vi "Build Report String.vi"(0 "folders":string[](array[string]), 5 "file paths":path[][](array[path]), 11 "error in":errorcluster) -> (4 "report string out":string, 15 "error out":errorcluster)   [LabVIEW 2019, in "MD Generator.lvlib"]
uses:
  MD Generator.lvlib
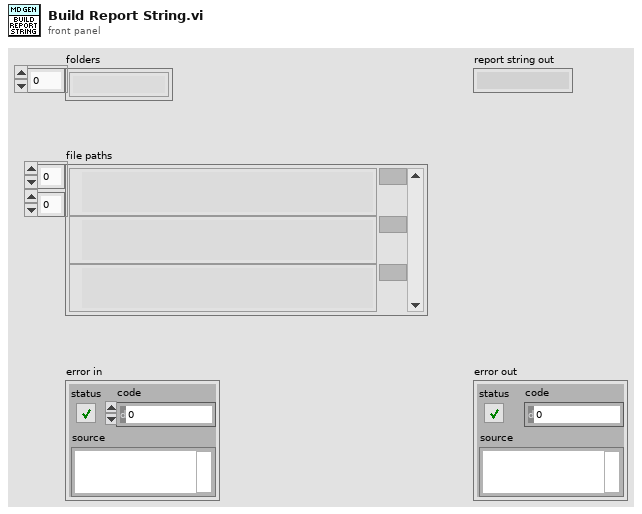
[diagram p1: front panel]
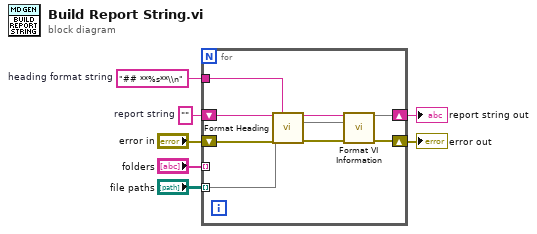
[diagram p0: block diagram]
diagram:
  w2 = ""  # report string
  w7 = "## **%s**\\n"  # heading format string
  n1 = for {
    shift-right: [w14] -> w1
    shift-left: w2 -> [w13]
    shift-right: [w12] -> w3
    shift-left: "error in" -> [w11]
    tunnel: w7 -> [w9]
    tunnel: "folders" -> [_] mode=indexing
    tunnel: "file paths" -> [w8] mode=indexing
    n2 = call "Format Heading.vi"("new heading"=w13, "format string"=w9, "error in"=w11) -> ("string out"=w10:string, "error out"=w15:errorcluster)  [unwired: 11 in]
    n3 = call "Format VI Information.vi"("filenames"=w10, 5:w8, "error in"=w15) -> (4:w14, "error out"=w12:errorcluster)  [unwired: 10 in, 1 out]
  }
  "error out" <- w3
  "report string out" <- w1
